vi "Get Feature Names.vi"(8 "error in (no error)":errorcluster caption="entrée d'erreur (pas d'erreur)", 9 "y":string[][](array[string]), 10 "X":string[][](array[string]), 11 "PolynomialFeatures.lvclass":refnum<class "PolynomialFeatures.lvclass">) -> (0 "error out":errorcluster caption="sortie d'erreur", 2 "Data":T1, 3 "PolynomialFeatures.lvclass":refnum<class "PolynomialFeatures.lvclass">)   [LabVIEW 2020, in "PolynomialFeatures.lvclass"]
doc: "Return feature names for output features\n\nReturns : \n\n- output_feature_names : list of string, length n_output_features"
uses:
  PolynomialFeatures.lvclass
  PolynomialFeatures.lvclass/PolynomialFeatures.ctl
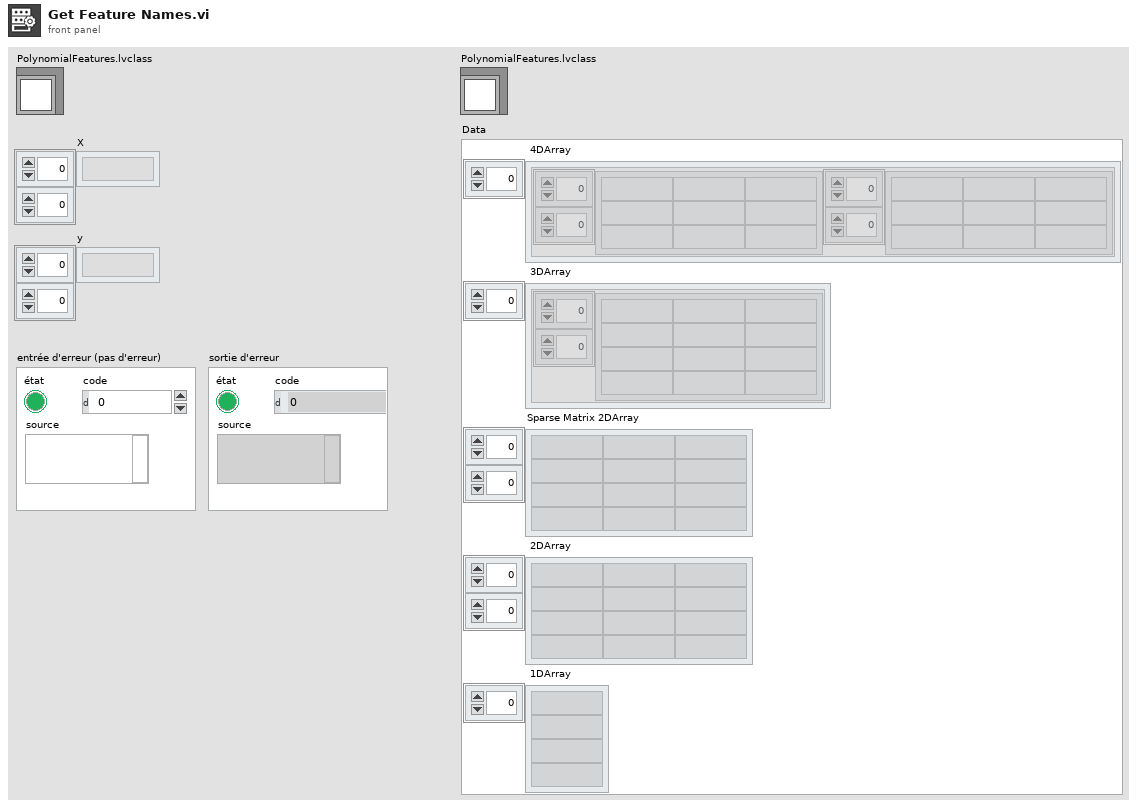
[diagram p1: front panel]
types:
  T1 = cluster{" 4DArray":cluster{"1":string[][], "2":string[][]}[], " 3DArray":cluster{"Tableau":string[][]}[], "Sparse Matrix 2DArray":string[][], " 2DArray":string[][], " 1DArray":string[]}
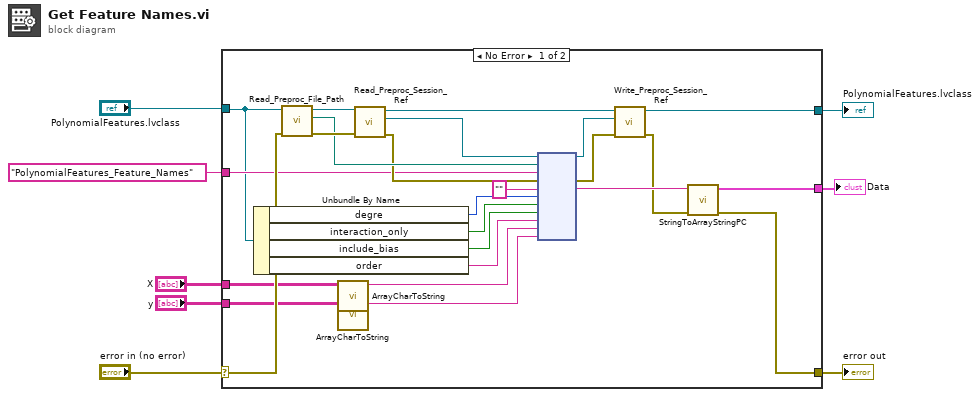
[diagram p0: block diagram]
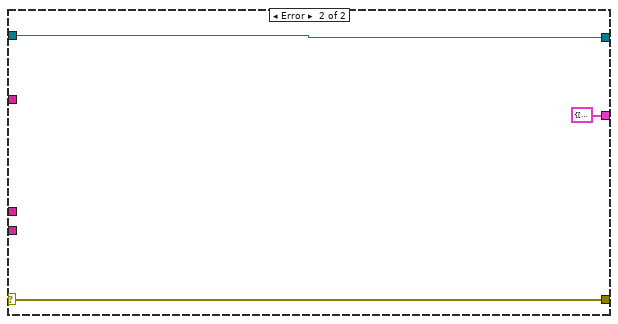
[diagram p2: hidden frame]
diagram:
  n1 = case shown="No Error" "error in (no error)" {
    selector: "error in (no error)" -> [w21 w36]
    tunnel: [w10 w36] -> w7
    tunnel: [w9 w35] -> w5
    tunnel: "PolynomialFeatures.lvclass" -> [w19 w35]
    tunnel: "PolynomialFeatures_Feature_Names" ("Fonction") -> [w20 _]
    tunnel: [w11 T1 {" 4DArray"=[], " 3DArray"=[], "Sparse Matrix 2DArray"=[], " 2DArray"=[], " 1DArray"=[]} ("Data")] -> w3
    tunnel: "X" -> [w17 _]
    tunnel: "y" -> [w15 _]
    frame No Error {
      n2 = Unbundle By Name(w19) -> ("degre"=w24:i32, "interaction_only"=w23:bool, "include_bias"=w22:bool, "order"=w18:string)
      n3 = call-dynamic "Read_Preproc_File_Path.vi"("error in (no error)"=w21, "Python in"=w19) -> ("error out"=w32:errorcluster, "File_Path"=w29:path, "Python out"=w33:refnum<class "PolynomialFeatures.lvclass">)  [unwired: 7 in]
      n4 = call "ArrayCharToString.vi"("TAB"=w17) -> ("Instruction"=w16:string)  [unwired: 10 in]
      n5 = call "ArrayCharToString.vi"("TAB"=w15) -> ("Instruction"=w14:string)  [unwired: 10 in]
      n6 = call-dynamic "Read_Preproc_Session_Ref.vi"("error in (no error)"=w32, "Python in"=w33) -> ("error out"=w28:errorcluster, "Session_ref"=w30:refnum<k35>, "Python out"=w31:refnum<class "PolynomialFeatures.lvclass">)  [unwired: 7 in]
      n7 = node(w30, w29, w20, w28, "", w24, w23, w22, w18, w16, w14) -> (w26:refnum<k35>, w27:errorcluster, w13:string)  [unwired: 6 in, 2 out]
      n8 = call-dynamic "Write_Preproc_Session_Ref.vi"("error in (no error)"=w27, "Session_ref"=w26, "Python in"=w31) -> ("error out"=w12:errorcluster, "Python out"=w9:refnum<class "PolynomialFeatures.lvclass">)  [unwired: 7 in]
      n9 = call "StringToArrayStringPC.vi"("sortie d'erreur"=w12, "Return value"=w13) -> ("sortie d'erreur"=w10:errorcluster, "Data"=w11:T1)  [unwired: 8 in]
    }
    frame Error {
    }
  }
  "error out" <- w7
  "PolynomialFeatures.lvclass" <- w5
  "Data" <- w3
